vi "Get Steering Angles.vi"(11 "Input Steering":T6) -> (3 "Steering Angles (deg)":T7)   [LabVIEW 2020]
doc: "takes in cluster of steering motors in <b>ticks</b> and returns a cluster of pod steering angles in <b>degrees"
uses:
  <vilib>/Rock Robotics/WPI/MotorControl/WPI_MotorControlDeviceRef.ctl
  <vilib>/Rock Robotics/WPI/MotorControl/WPI_MotorControlType.ctl
  <vilib>/Rock Robotics/SystemInterfaces/DIO/FPGA_DIOPWMChannel.ctl
  <vilib>/Rock Robotics/WPI/PWM/WPI_PWMDeadband.ctl
  <vilib>/Rock Robotics/SystemInterfaces/DIO/FPGA_DIOChannel.ctl
  <vilib>/Rock Robotics/WPI/ThirdParty/Phoenix-LabVIEW/Motor Controller/Get/CTRE_Phoenix_MotorController_GetSelectedSensorData.vi
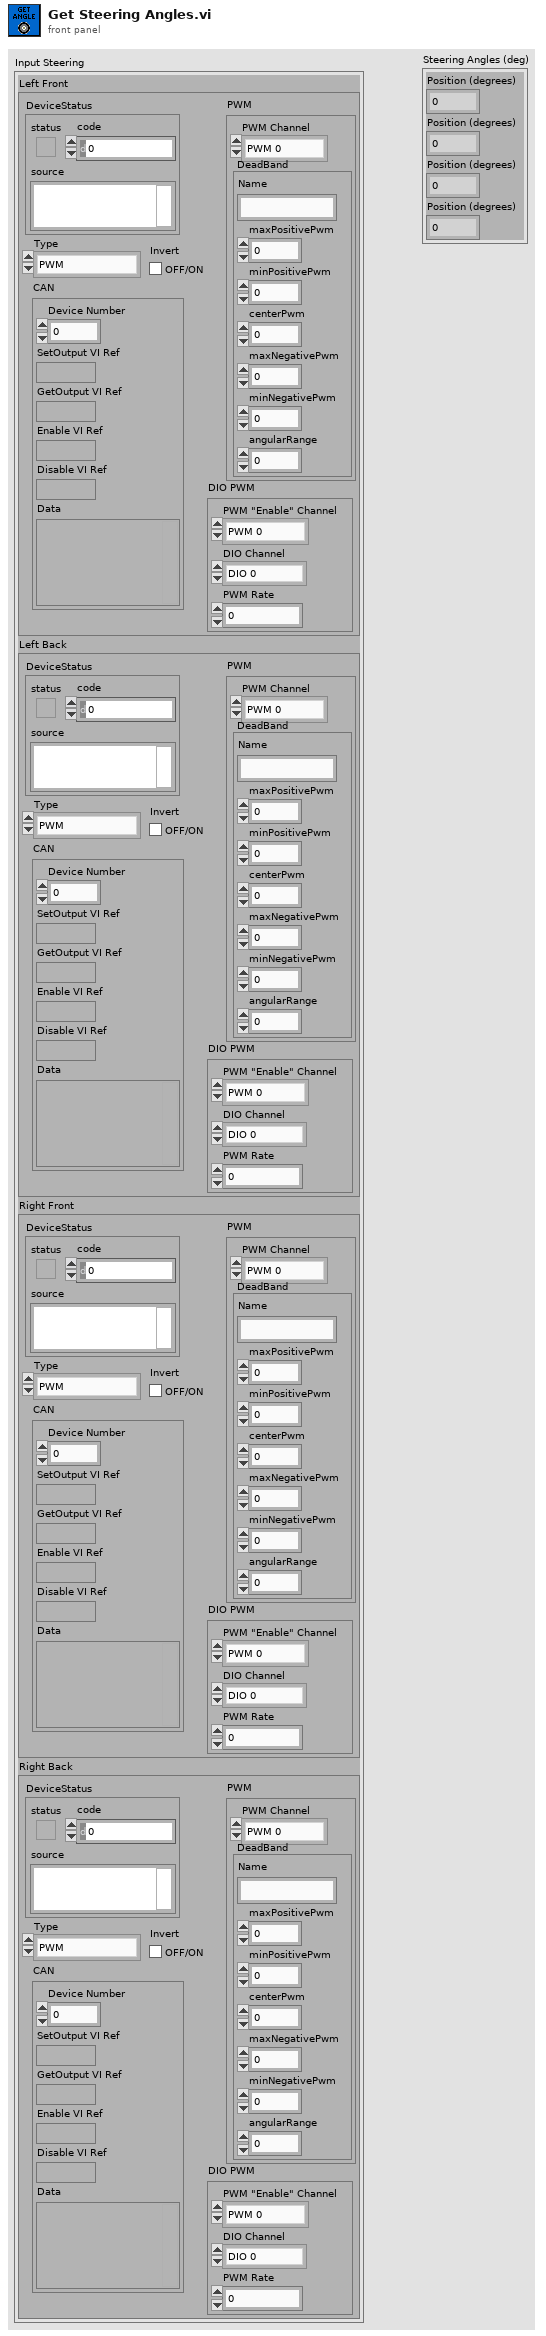
[diagram p1: front panel]
types:
  T1 = typedef "WPI_MotorControlDeviceRef.ctl" = cluster{"DeviceStatus":errorcluster, "Type":T2, "PWM":cluster{"PWM Channel":T3, "DeadBand":T4}, "CAN":cluster{"Device Number":u8, "SetOutput VI Ref":variant, "GetOutput VI Ref":variant, "Enable VI Ref":variant, "Disable VI Ref":variant, "Data":variant}, "Invert":bool, "DIO PWM":cluster{"PWM \"Enable\" Channel":T3, "DIOChannel":T5, "PWM Rate":dbl}}
  T2 = typedef "WPI_MotorControlType.ctl" = enum16{"PWM", "CAN", "DIO PWM"}
  T3 = typedef "FPGA_DIOPWMChannel.ctl" = enum8{"PWM 0", "PWM 1", "PWM 2", "PWM 3", "PWM 4", "PWM 5", "PWM 6", "PWM 7", "PWM 8", "PWM 9", "PWM MXP 0", "PWM MXP 1", "PWM MXP 2", "PWM MXP 3", "PWM MXP 4", "PWM MXP 5", "PWM MXP 6", "PWM MXP 7", "PWM MXP 8", "PWM MXP 9", "Invalid"}
  T4 = typedef "WPI_PWMDeadband.ctl" = cluster{"Name":string, "maxPositivePwm":i32, "minPositivePwm":i32, "centerPwm":i32, "maxNegativePwm":i32, "minNegativePwm":i32, "angularRange":u16}
  T5 = typedef "FPGA_DIOChannel.ctl" = enum8{"DIO 0", "DIO 1", "DIO 2", "DIO 3", "DIO 4", "DIO 5", "DIO 6", "DIO 7", "DIO 8", "DIO 9", "DIO MXP 0", "DIO MXP 1", "DIO MXP 2", "DIO MXP 3", "DIO MXP 4", "DIO MXP 5", "DIO MXP 6", "DIO MXP 7", "DIO MXP 8", "DIO MXP 9", "DIO MXP 10", "DIO MXP 11", "DIO MXP 12", "DIO MXP 13", "DIO MXP 14", "DIO MXP 15", "SPI Port CS1", "SPI Port CS2", "SPI Port CS3", "SPI Port MISO", "SPI Port MOSI", "Invalid"}
  T6 = cluster{"Left Front":T1, "Left Back":T1, "Right Front":T1, "Right Back":T1}
  T7 = cluster{"Position (degrees)":dbl, "Position (degrees)":dbl, "Position (degrees)":dbl, "Position (degrees)":dbl}
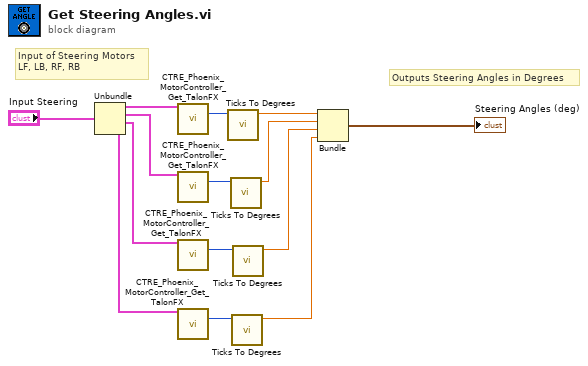
[diagram p0: block diagram]
diagram:
  # "Outputs Steering Angles in Degrees"
  # "Input of Steering Motors\nLF, LB, RF, RB"
  n1 = Unbundle("Input Steering") -> ("Left Front"=w9:T1, "Left Back"=w8:T1, "Right Front"=w7:T1, "Right Back"=w6:T1)
  n2 = call-poly <vilib>:"CTRE_Phoenix_MotorController_Get_TalonFX.vi"("PhoenixMotorControlDevRef"=w9) -> ("Position (Raw Sensor Units)"=w11:i32)  [unwired: 11 in, 3 out]
  n3 = call-poly <vilib>:"CTRE_Phoenix_MotorController_Get_TalonFX.vi"("PhoenixMotorControlDevRef"=w8) -> ("Position (Raw Sensor Units)"=w12:i32)  [unwired: 11 in, 3 out]
  n4 = call-poly <vilib>:"CTRE_Phoenix_MotorController_Get_TalonFX.vi"("PhoenixMotorControlDevRef"=w7) -> ("Position (Raw Sensor Units)"=w13:i32)  [unwired: 11 in, 3 out]
  n5 = call-poly <vilib>:"CTRE_Phoenix_MotorController_Get_TalonFX.vi"("PhoenixMotorControlDevRef"=w6) -> ("Position (Raw Sensor Units)"=w14:i32)  [unwired: 11 in, 3 out]
  n6 = call "Ticks To Degrees.vi"("Position (ticks)"=w11) -> ("Position (degrees)"=w5:dbl)  [unwired: 10 in]
  n7 = call "Ticks To Degrees.vi"("Position (ticks)"=w12) -> ("Position (degrees)"=w4:dbl)  [unwired: 10 in]
  n8 = call "Ticks To Degrees.vi"("Position (ticks)"=w14) -> ("Position (degrees)"=w2:dbl)  [unwired: 10 in]
  n9 = call "Ticks To Degrees.vi"("Position (ticks)"=w13) -> ("Position (degrees)"=w3:dbl)  [unwired: 10 in]
  n10 = Bundle("Position (degrees)"=w5, "Position (degrees)"=w4, "Position (degrees)"=w3, "Position (degrees)"=w2) -> (→"Steering Angles (deg)":T7)  [unwired: 1 in]
